vi "CRYSet Digital IO Setting Front Panel.vi"(11 "Vi Ref":refnum<vi>) -> ()   [LabVIEW 2013]
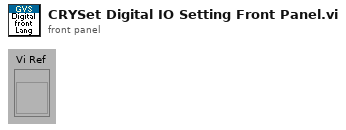
[diagram p1: front panel]
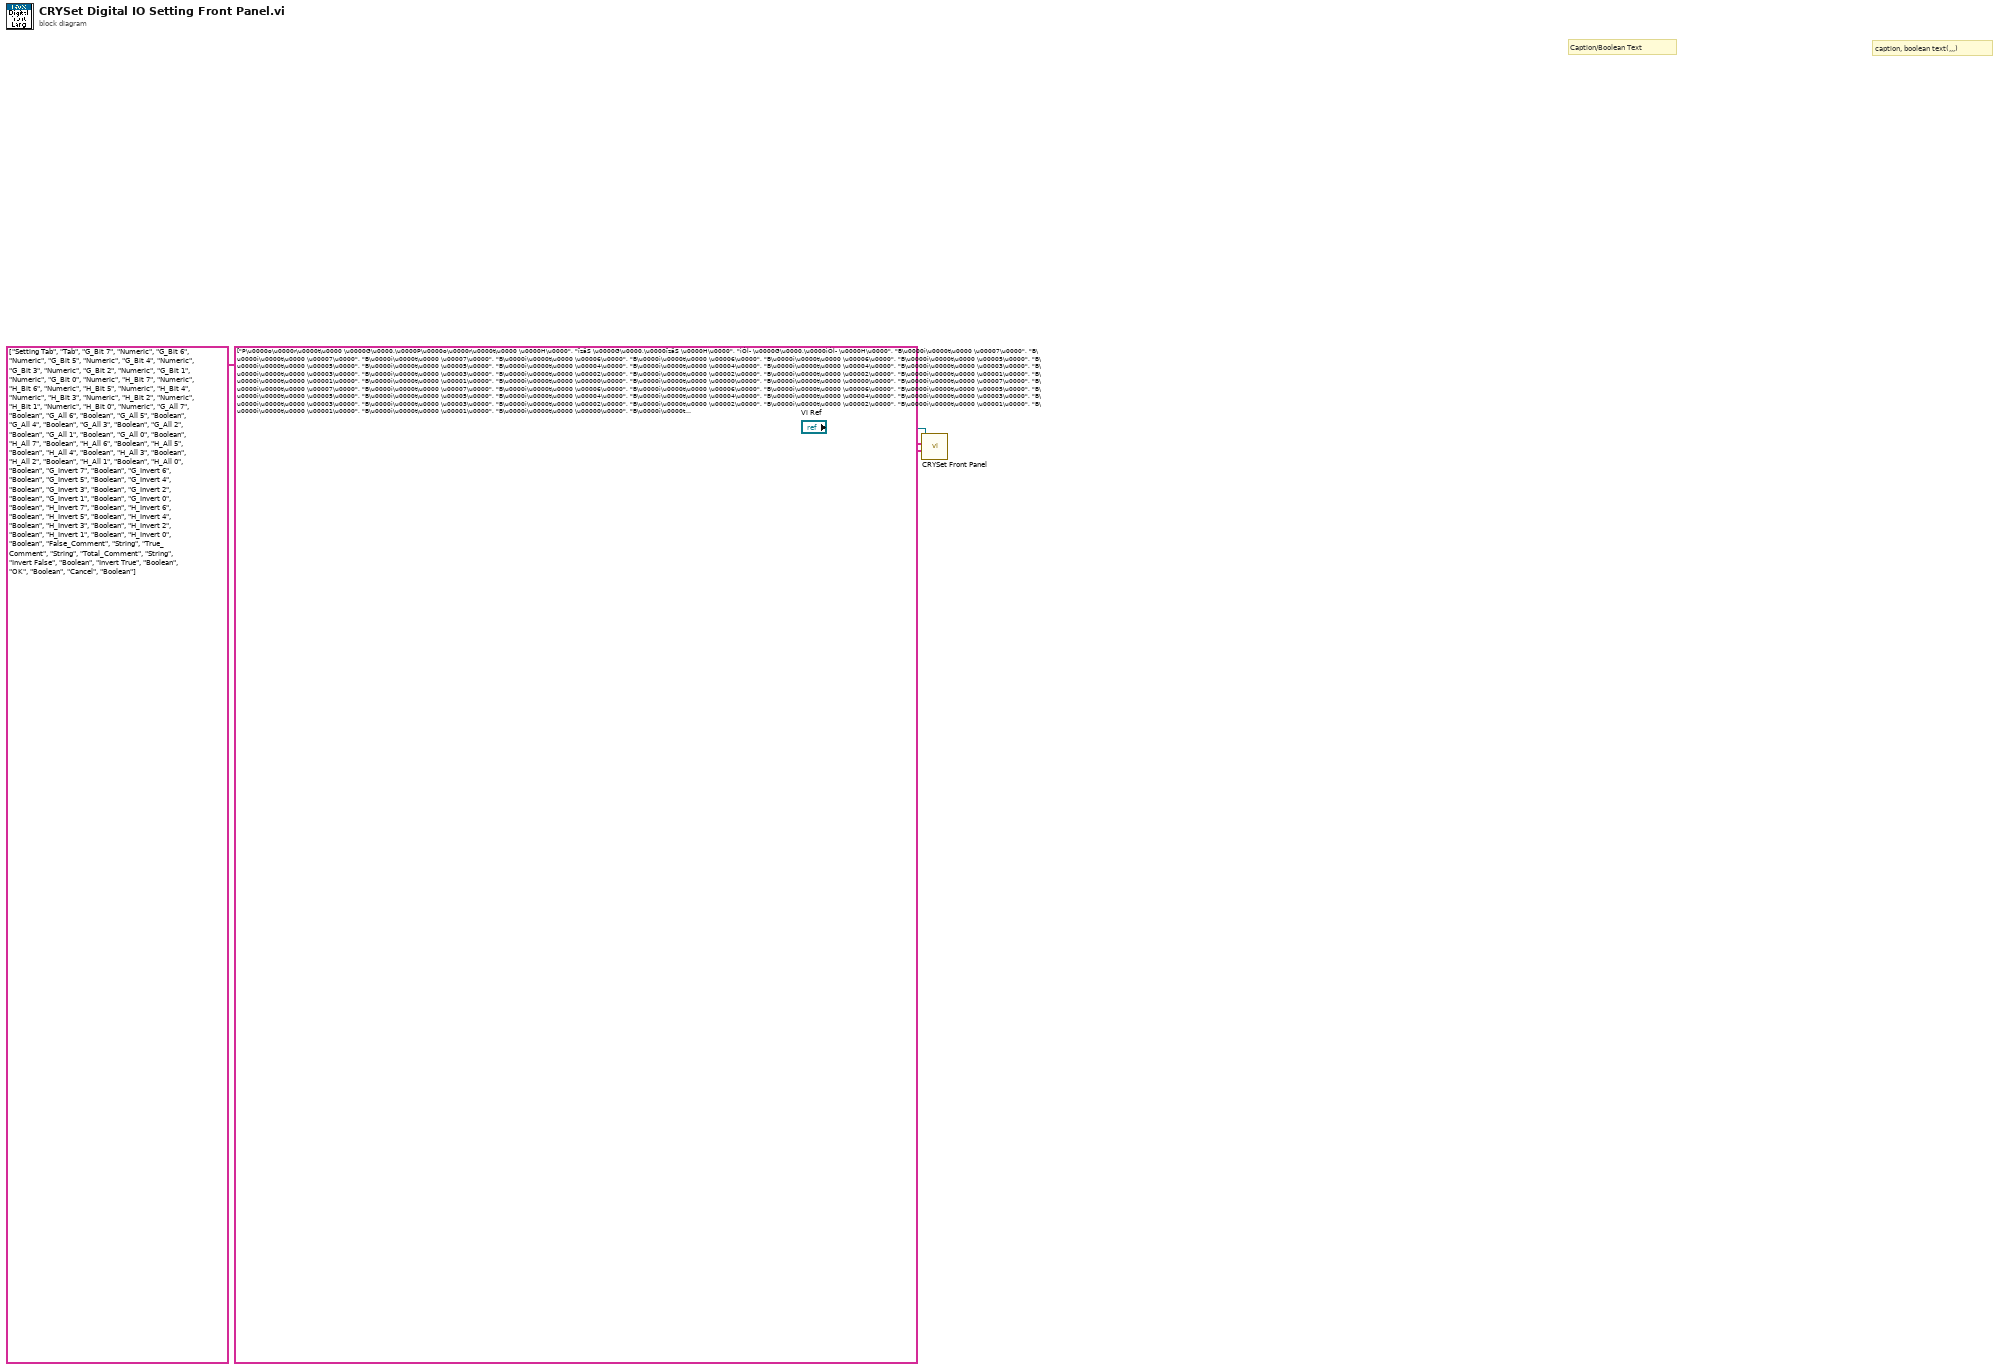
[diagram p0: block diagram]
diagram:
  # "Caption, Tab Page, Multilist Header, Button 4"
  # "Control Type"
  # "Control Name and Tab"
  # "caption, boolean text(,,,)"
  # "Caption/Boolean Text"
  n1 = call "CRYSet Front Panel.vi"("Caption(Boolean Text)"=string[][] [["P\u0000o\u0000r\u0000t\u0000 \u0000G\u0000,\u0000P\u0000o\u0000r\u0000t\u0000 \u0000H\u0000", "ïzãS \u0000G\u0000,\u0000ïzãS \u0000H\u0000", "ìÓl­ \u0000G\u0000,\u0000ìÓl­ \u0000H\u0000"], ["B\u0000i\u0000t\u0000 \u00007\u0000", "B\u0000i\u0000t\u0000 \u00007\u0000", "B\u0000i\u0000t\u0000 \u00007\u0000"], ["B\u0000i\u0000t\u0000 \u00006\u0000", "B\u0000i\u0000t\u0000 \u00006\u0000", "B\u0000i\u0000t\u0000 \u00006\u0000"], ["B\u0000i\u0000t\u0000 \u00005\u0000", "B\u0000i\u0000t\u0000 \u00005\u0000", "B\u0000i\u0000t\u0000 \u00005\u0000"], ["B\u0000i\u0000t\u0000 \u00004\u0000", "B\u0000i\u0000t\u0000 \u00004\u0000", "B\u0000i\u0000t\u0000 \u00004\u0000"], ["B\u0000i\u0000t\u0000 \u00003\u0000", "B\u0000i\u0000t\u0000 \u00003\u0000", "B\u0000i\u0000t\u0000 \u00003\u0000"], ["B\u0000i\u0000t\u0000 \u00002\u0000", "B\u0000i\u0000t\u0000 \u00002\u0000", "B\u0000i\u0000t\u0000 \u00002\u0000"], ["B\u0000i\u0000t\u0000 \u00001\u0000", "B\u0000i\u0000t\u0000 \u00001\u0000", "B\u0000i\u0000t\u0000 \u00001\u0000"], ["B\u0000i\u0000t\u0000 \u00000\u0000", "B\u0000i\u0000t\u0000 \u00000\u0000", "B\u0000i\u0000t\u0000 \u00000\u0000"], ["B\u0000i\u0000t\u0000 \u00007\u0000", "B\u0000i\u0000t\u0000 \u00007\u0000", "B\u0000i\u0000t\u0000 \u00007\u0000"], ["B\u0000i\u0000t\u0000 \u00006\u0000", "B\u0000i\u0000t\u0000 \u00006\u0000", "B\u0000i\u0000t\u0000 \u00006\u0000"], ["B\u0000i\u0000t\u0000 \u00005\u0000", "B\u0000i\u0000t\u0000 \u00005\u0000", "B\u0000i\u0000t\u0000 \u00005\u0000"], ["B\u0000i\u0000t\u0000 \u00004\u0000", "B\u0000i\u0000t\u0000 \u00004\u0000", "B\u0000i\u0000t\u0000 \u00004\u0000"], ["B\u0000i\u0000t\u0000 \u00003\u0000", "B\u0000i\u0000t\u0000 \u00003\u0000", "B\u0000i\u0000t\u0000 \u00003\u0000"], ["B\u0000i\u0000t\u0000 \u00002\u0000", "B\u0000i\u0000t\u0000 \u00002\u0000", "B\u0000i\u0000t\u0000 \u00002\u0000"], ["B\u0000i\u0000t\u0000 \u00001\u0000", "B\u0000i\u0000t\u0000 \u00001\u0000", "B\u0000i\u0000t\u0000 \u00001\u0000"], ["B\u0000i\u0000t\u0000 \u00000\u0000", "B\u0000i\u0000t\u0000 \u00000\u0000", "B\u0000i\u0000t\u0000 \u00000\u0000"], ["A\u0000l\u0000l\u0000", "@b\tg", "\u0004È´Ì"], ["A\u0000l\u0000l\u0000", "@b\tg", "\u0004È´Ì"], ["A\u0000l\u0000l\u0000", "@b\tg", "\u0004È´Ì"], ["A\u0000l\u0000l\u0000", "@b\tg", "\u0004È´Ì"], ["A\u0000l\u0000l\u0000", "@b\tg", "\u0004È´Ì"], ["A\u0000l\u0000l\u0000", "@b\tg", "\u0004È´Ì"], ["A\u0000l\u0000l\u0000", "@b\tg", "\u0004È´Ì"], ["A\u0000l\u0000l\u0000", "@b\tg", "\u0004È´Ì"], ["A\u0000l\u0000l\u0000", "@b\tg", "\u0004È´Ì"], ["A\u0000l\u0000l\u0000", "@b\tg", "\u0004È´Ì"], ["A\u0000l\u0000l\u0000", "@b\tg", "\u0004È´Ì"], ["A\u0000l\u0000l\u0000", "@b\tg", "\u0004È´Ì"], ["A\u0000l\u0000l\u0000", "@b\tg", "\u0004È´Ì"], ["A\u0000l\u0000l\u0000", "@b\tg", "\u0004È´Ì"], ["A\u0000l\u0000l\u0000", "@b\tg", "\u0004È´Ì"], ["A\u0000l\u0000l\u0000", "@b\tg", "\u0004È´Ì"], ["I\u0000n\u0000v\u0000e\u0000r\u0000t\u0000", "úQÍSl", "œÍl­\u0018¼\u0004È"], ["I\u0000n\u0000v\u0000e\u0000r\u0000t\u0000", "úQÍSl", "œÍl­\u0018¼\u0004È"], ["I\u0000n\u0000v\u0000e\u0000r\u0000t\u0000", "úQÍSl", "œÍl­\u0018¼\u0004È"], ["I\u0000n\u0000v\u0000e\u0000r\u0000t\u0000", "úQÍSl", "œÍl­\u0018¼\u0004È"], ["I\u0000n\u0000v\u0000e\u0000r\u0000t\u0000", "úQÍSl", "œÍl­\u0018¼\u0004È"], ["I\u0000n\u0000v\u0000e\u0000r\u0000t\u0000", "úQÍSl", "œÍl­\u0018¼\u0004È"], ["I\u0000n\u0000v\u0000e\u0000r\u0000t\u0000", "úQÍSl", "œÍl­\u0018¼\u0004È"], ["I\u0000n\u0000v\u0000e\u0000r\u0000t\u0000", "úQÍSl", "œÍl­\u0018¼\u0004È"], ["I\u0000n\u0000v\u0000e\u0000r\u0000t\u0000", "úQÍSl", "œÍl­\u0018¼\u0004È"], ["I\u0000n\u0000v\u0000e\u0000r\u0000t\u0000", "úQÍSl", "œÍl­\u0018¼\u0004È"], ["I\u0000n\u0000v\u0000e\u0000r\u0000t\u0000", "úQÍSl", "œÍl­\u0018¼\u0004È"], ["I\u0000n\u0000v\u0000e\u0000r\u0000t\u0000", "úQÍSl", "œÍl­\u0018¼\u0004È"], ["I\u0000n\u0000v\u0000e\u0000r\u0000t\u0000", "úQÍSl", "œÍl­\u0018¼\u0004È"], ["I\u0000n\u0000v\u0000e\u0000r\u0000t\u0000", "úQÍSl", "œÍl­\u0018¼\u0004È"], ["I\u0000n\u0000v\u0000e\u0000r\u0000t\u0000", "úQÍSl", "œÍl­\u0018¼\u0004È"], ["I\u0000n\u0000v\u0000e\u0000r\u0000t\u0000", "úQÍSl", "œÍl­\u0018¼\u0004È"], ["F\u0000a\u0000l\u0000s\u0000e\u0000_\u0000C\u0000o\u0000m\u0000m\u0000e\u0000n\u0000t\u0000,\u0000 \u0000T\u0000r\u0000u\u0000e\u0000 \u0000=\u0000 \u0000O\u0000n\u0000 \u0000 \u0000 \u0000 \u0000 \u0000F\u0000a\u0000l\u0000s\u0000e\u0000 \u0000=\u0000 \u0000O\u0000f\u0000f\u0000", "F\u0000a\u0000l\u0000s\u0000e\u0000_\u0000C\u0000o\u0000m\u0000m\u0000e\u0000n\u0000t\u0000,\u0000 \u0000\u001fw \u0000=\u0000 \u0000¥c \u0000 \u0000 \u0000 \u0000 \u0000GP \u0000=\u0000 \u0000­e", "F\u0000a\u0000l\u0000s\u0000e\u0000_\u0000C\u0000o\u0000m\u0000m\u0000e\u0000n\u0000t\u0000,\u00008Ì \u0000=\u0000 \u0000\u001cÏ0® \u0000 \u0000 \u0000 \u0000 \u0000p¬ÓÉ \u0000=\u0000 \u0000D°0®"], ["T\u0000r\u0000u\u0000e\u0000_\u0000C\u0000o\u0000m\u0000m\u0000e\u0000n\u0000t\u0000,\u0000 \u0000T\u0000r\u0000u\u0000e\u0000 \u0000=\u0000 \u0000O\u0000f\u0000f\u0000 \u0000 \u0000 \u0000 \u0000 \u0000F\u0000a\u0000l\u0000s\u0000e\u0000 \u0000=\u0000 \u0000O\u0000n\u0000", "T\u0000r\u0000u\u0000e\u0000_\u0000C\u0000o\u0000m\u0000m\u0000e\u0000n\u0000t\u0000,\u0000 \u0000\u001fw \u0000=\u0000 \u0000­e \u0000 \u0000 \u0000 \u0000 \u0000GP \u0000=\u0000 \u0000¥c", "T\u0000r\u0000u\u0000e\u0000_\u0000C\u0000o\u0000m\u0000m\u0000e\u0000n\u0000t\u0000,\u00008Ì \u0000=\u0000 \u0000D°0® \u0000 \u0000 \u0000 \u0000 \u0000p¬ÓÉ \u0000=\u0000 \u0000\u001cÏ0®"], ["T\u0000o\u0000t\u0000a\u0000l\u0000_\u0000C\u0000o\u0000m\u0000m\u0000e\u0000n\u0000t\u0000,\u0000 \u0000T\u0000h\u0000e\u0000 \u0000r\u0000e\u0000s\u0000u\u0000l\u0000t\u0000s\u0000 \u0000a\u0000r\u0000e\u0000 \u0000\"\u0000B\u0000o\u0000o\u0000l\u0000e\u0000a\u0000n\u0000 \u0000A\u0000n\u0000d\u0000\"\u0000 \u0000o\u0000f\u0000 \u0000i\u0000t\u0000e\u0000m\u0000s\u0000 \u0000s\u0000e\u0000l\u0000e\u0000c\u0000t\u0000e\u0000d\u0000.\u0000", "T\u0000o\u0000t\u0000a\u0000l\u0000_\u0000C\u0000o\u0000m\u0000m\u0000e\u0000n\u0000t\u0000,\u0000Ó~g/f«\tébvyîvv\"\u0000\u0003^\u0014\\XN\"\u0000.\u0000", "T\u0000o\u0000t\u0000a\u0000l\u0000_\u0000C\u0000o\u0000m\u0000m\u0000e\u0000n\u0000t\u0000,\u0000°¬ü¬”² \u0000 ÁÝÐ\u001c´ \u0000mÕ©ºä´XÇ \u0000\"\u0000`¸¬¹\u0001È\"\u0000…ÇÈ²ä².\u0000"], ["I\u0000n\u0000v\u0000e\u0000r\u0000t\u0000", "úQÍSl", "œÍl­\u0018¼\u0004È"], ["I\u0000n\u0000v\u0000e\u0000r\u0000t\u0000", "úQÍSl", "œÍl­\u0018¼\u0004È"], ["O\u0000K\u0000", "nx¤‹", "UÖxÇ"], ["C\u0000a\u0000n\u0000c\u0000e\u0000l\u0000", "ÖSˆm", "èÍŒÁ"]], "Control ID and Type(Label Name, Type)"=string[][] [["Setting Tab", "Tab"], ["G_Bit 7", "Numeric"], ["G_Bit 6", "Numeric"], ["G_Bit 5", "Numeric"], ["G_Bit 4", "Numeric"], ["G_Bit 3", "Numeric"], ["G_Bit 2", "Numeric"], ["G_Bit 1", "Numeric"], ["G_Bit 0", "Numeric"], ["H_Bit 7", "Numeric"], ["H_Bit 6", "Numeric"], ["H_Bit 5", "Numeric"], ["H_Bit 4", "Numeric"], ["H_Bit 3", "Numeric"], ["H_Bit 2", "Numeric"], ["H_Bit 1", "Numeric"], ["H_Bit 0", "Numeric"], ["G_All 7", "Boolean"], ["G_All 6", "Boolean"], ["G_All 5", "Boolean"], ["G_All 4", "Boolean"], ["G_All 3", "Boolean"], ["G_All 2", "Boolean"], ["G_All 1", "Boolean"], ["G_All 0", "Boolean"], ["H_All 7", "Boolean"], ["H_All 6", "Boolean"], ["H_All 5", "Boolean"], ["H_All 4", "Boolean"], ["H_All 3", "Boolean"], ["H_All 2", "Boolean"], ["H_All 1", "Boolean"], ["H_All 0", "Boolean"], ["G_Invert 7", "Boolean"], ["G_Invert 6", "Boolean"], ["G_Invert 5", "Boolean"], ["G_Invert 4", "Boolean"], ["G_Invert 3", "Boolean"], ["G_Invert 2", "Boolean"], ["G_Invert 1", "Boolean"], ["G_Invert 0", "Boolean"], ["H_Invert 7", "Boolean"], ["H_Invert 6", "Boolean"], ["H_Invert 5", "Boolean"], ["H_Invert 4", "Boolean"], ["H_Invert 3", "Boolean"], ["H_Invert 2", "Boolean"], ["H_Invert 1", "Boolean"], ["H_Invert 0", "Boolean"], ["False_Comment", "String"], ["True_Comment", "String"], ["Total_Comment", "String"], ["Invert False", "Boolean"], ["Invert True", "Boolean"], ["OK", "Boolean"], ["Cancel", "Boolean"]], "Vi Ref"="Vi Ref") -> ()  [unwired: 9 in]
